vi "DAQ Initialize.vi"(0 "MCC USB-DAQ Setup":T1 {"Voltage Monitor"."Input Voltage Range" items=["+/-10 V Range", "+/-5 V Range", "+/-2.5V Range", "+/-1.25 V Range", "+/-0.625 V Range", "+/-0.3125 V Range", "+/-0.1562V Range", "+/-0.078125 V Range"]; "Aux Sensor 3/EC"."Input Voltage Range" items=["+/-10 V Range", "+/-5 V Range", "+/-2.5V Range", "+/-1.25 V Range", "+/-0.625 V Range", "+/-0.3125 V Range", "+/-0.1562V Range", "+/-0.078125 V Range"]; "Aux Sensor 2"."Input Voltage Range" items=["+/-10 V Range", "+/-5 V Range", "+/-2.5V Range", "+/-1.25 V Range", "+/-0.625 V Range", "+/-0.3125 V Range", "+/-0.1562V Range", "+/-0.078125 V Range"]; "Aux Sensor 1"."Input Voltage Range" items=["+/-10 V Range", "+/-5 V Range", "+/-2.5V Range", "+/-1.25 V Range", "+/-0.625 V Range", "+/-0.3125 V Range", "+/-0.1562V Range", "+/-0.078125 V Range"]; "String Pot Signal"."Input Voltage Range" items=["+/-10 V Range", "+/-5 V Range", "+/-2.5V Range", "+/-1.25 V Range", "+/-0.625 V Range", "+/-0.3125 V Range", "+/-0.1562V Range", "+/-0.078125 V Range"]; "Top String Pot"."Input Voltage Range" items=["+/-10 V Range", "+/-5 V Range", "+/-2.5V Range", "+/-1.25 V Range", "+/-0.625 V Range", "+/-0.3125 V Range", "+/-0.1562V Range", "+/-0.078125 V Range"]; "DHT Pressure Sensor"."Input Voltage Range" items=["+/-10 V Range", "+/-5 V Range", "+/-2.5V Range", "+/-1.25 V Range", "+/-0.625 V Range", "+/-0.3125 V Range", "+/-0.1562V Range", "+/-0.078125 V Range"]; "McMillian 102 Flowmeter"."Input Voltage Range" items=["+/-10 V Range", "+/-5 V Range", "+/-2.5V Range", "+/-1.25 V Range", "+/-0.625 V Range", "+/-0.3125 V Range", "+/-0.1562V Range", "+/-0.078125 V Range"]; "Omega Pressure Sensor"."Input Voltage Range" items=["+/-10 V Range", "+/-5 V Range", "+/-2.5V Range", "+/-1.25 V Range", "+/-0.625 V Range", "+/-0.3125 V Range", "+/-0.1562V Range", "+/-0.078125 V Range"]}, 5 "DAQ \nData Rate S/s":dbl, 11 "error in (no error)":errorcluster) -> (1 "Array 2":string[](array[string]), 2 "Array":refnum<k24>[](array[refnum]), 3 "delimited string":string, 4 "Descriptions":string[](array[string]), 6 "Boolean":bool, 8 "Number of Channels":i32, 10 "Voltage Range":dbl[](array[numeric]), 13 "9V Voltage Monitor":dbl, 14 "Rate":dbl, 15 "error out":errorcluster)   [LabVIEW 2016]
uses:
  C:/Cascade-lv16-64/builds/Waterloo Main Program/cascade/data/ULx_LV.dll
  builds/Waterloo Main Program/cascade/data/ULx_LV.dll
  controls/MCC DAQ Setup.ctl
  controls/Aux Sensor.ctl
  <vilib>/ULx/Create Channel.llb/ULx Create Channel (AI-Voltage-Basic).vi
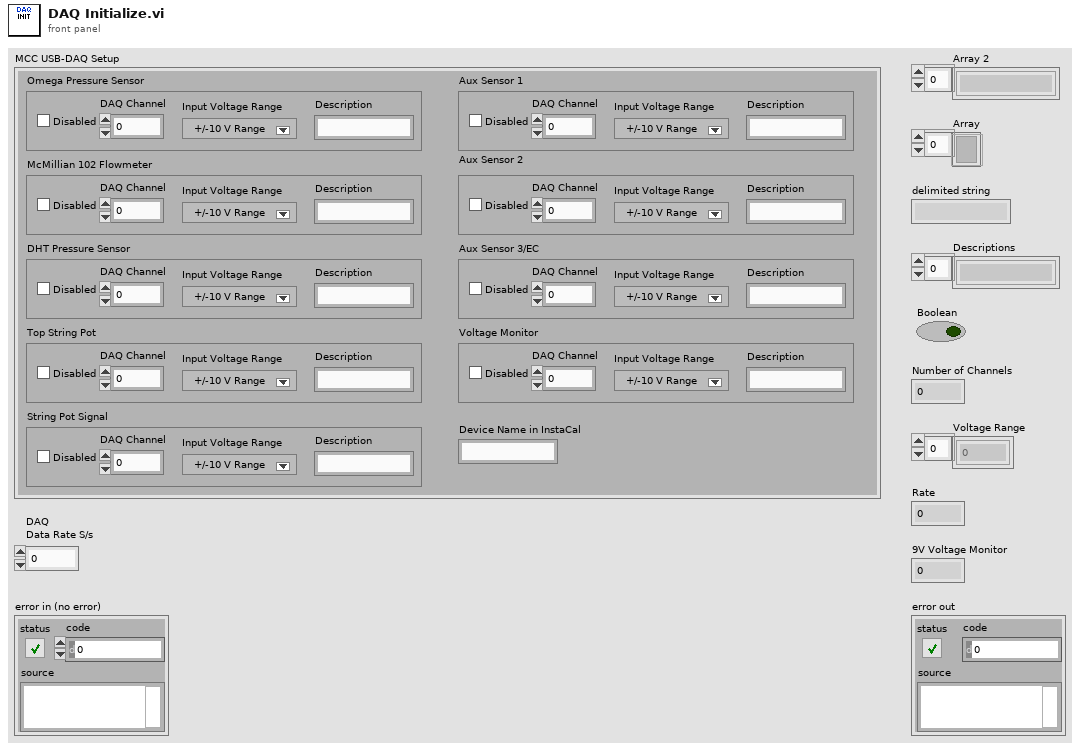
[diagram p1: front panel]
types:
  T1 = typedef "MCC DAQ Setup.ctl" = cluster{"Device Name in InstaCal":string, "Omega Pressure Sensor":T2, "McMillian 102 Flowmeter":T2, "DHT Pressure Sensor":T2, "Top String Pot":T2, "String Pot Signal":T2, "Aux Sensor 1":T2, "Aux Sensor 2":T2, "Aux Sensor 3/EC":T2, "Voltage Monitor":T2}
  T2 = typedef "Aux Sensor.ctl" = cluster{"DAQ Channel":dbl, "Input Voltage Range":u16, "Enabled":bool, "Description":string}
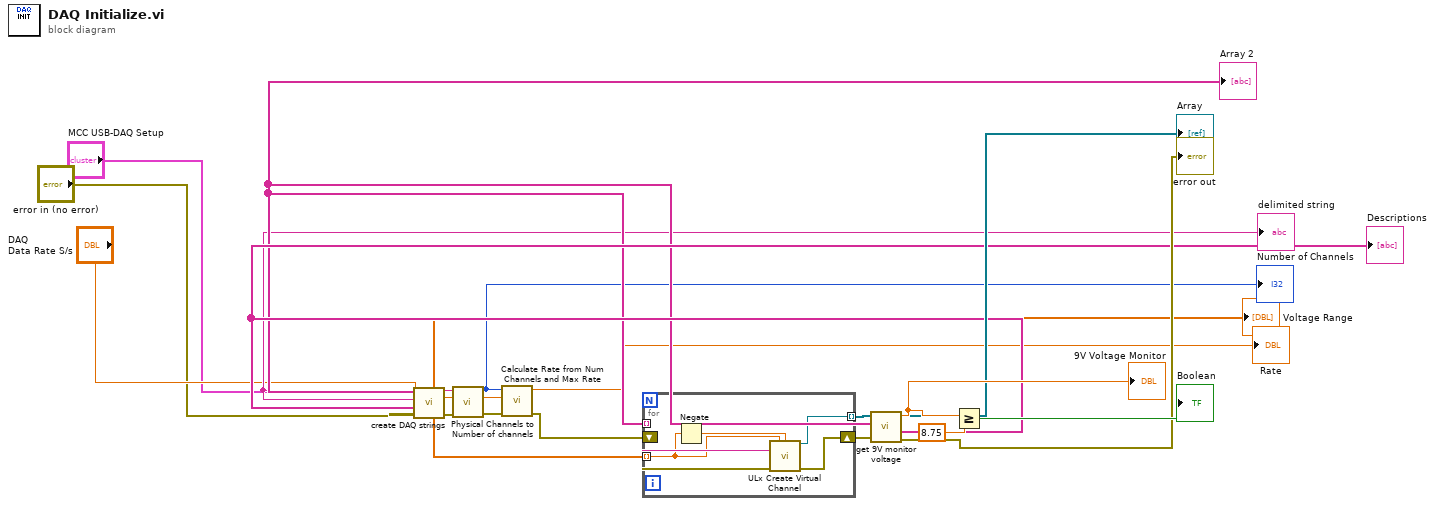
[diagram p0: block diagram]
diagram:
  n1 = call "create DAQ strings.vi"("error in (no error)"="error in (no error)", "MCC USB-DAQ Setup"="MCC USB-DAQ Setup") -> ("error IO"=w9:errorcluster, "Descriptions"=w11:string[], "delimited string"=w8:string, "Array"=w10:string[], "Voltage Range"=w3:dbl[])  [unwired: 5 in]
  "Descriptions" <- w11
  "Array 2" <- w10
  "delimited string" <- w8
  "Voltage Range" <- w3
  n2 = call "Physical Channels to Number of channels.vi"("error in (no error)"=w9, "Physical Channel in"=w8) -> ("error out"=w7:errorcluster, "Number of Channels"=w5:i32)  [unwired: 7 in, 1 out]
  "Number of Channels" <- w5
  n3 = call "Calculate Rate from Num Channels and Max Rate.vi"("error in (no error)"=w7, "Channel Data Rate S/s"="DAQ \nData Rate S/s", "Number of Channels"=w5) -> ("error out"=w12:errorcluster, "Rate"=→"Rate":dbl)  [unwired: 7 in]
  n4 = for {
    tunnel: w10 -> [w24] mode=indexing
    tunnel: w3 -> [w23] mode=indexing
    tunnel: [w20] -> w13 mode=indexing
    shift-right: [w21] -> w14
    shift-left: w12 -> [w19]
    n5 = Negate(x=w23) -> (-x=w22:dbl)
    n6 = call-poly <vilib>:"ULx Create Virtual Channel.vi"("maximum value"=w23, "minimum value"=w22, "physical channels"=w24, "error in"=w19) -> ("task out"=w20:refnum<k24>, "error out"=w21:errorcluster)  [unwired: 10 in]
  }
  "Array" <- w13
  n7 = call "get 9V monitor voltage.vi"("error in (no error)"=w14, "Descriptions"=w11, "Array"=w10, "Array 2"=w13) -> ("error out"=→"error out":errorcluster, "9V Voltage Monitor"=w16:dbl)  [unwired: 6 in]
  "9V Voltage Monitor" <- w16
  n8 = Greater Or Equal?(x=w16, y=8.75) -> (x >= y?=→"Boolean":bool)
